vi "FL_DEC_split_3_and_prefilter_(online).vi"(0 "DEC input cluster":T4, 1 "Pre-filter params.":T1, 2 "Initialize? (F)":bool) -> (3 "Times":T3, 4 "TTLs":cluster{"TTL input":i16, "TTL output":i16}, 5 "Magnets coords":cluster{"X1":dbl, "Y1":dbl, "X2":dbl, "Y2":dbl}, 6 "Magnets coords raw":T2)   [LabVIEW 2018, in "Tracker.lvlib"]
uses:
  Tracker.lvlib
  Controls/CTL_Decoded_data_frame.ctl
  Controls/CTL_Pre-filter_params.ctl
  <vilib>/ptbypt/NI_PtbyPt.lvlib
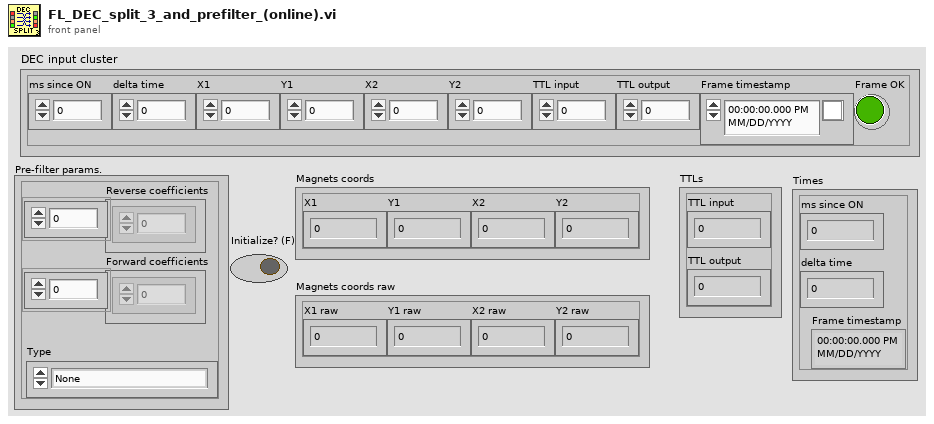
[diagram p1: front panel]
types:
  T1 = typedef "Tracker.lvlib/CTL_Pre-filter_params.ctl" = cluster{"Reverse coefficients":dbl[], "Forward coefficients":dbl[], "Type":enum16{"None", "FIR (PtbyPt)", "IIR (PtbyPt)"}}
  T2 = cluster{"X1 raw":dbl, "Y1 raw":dbl, "X2 raw":dbl, "Y2 raw":dbl}
  T3 = cluster{"ms since ON":u32, "delta time":u32, "Frame timestamp":timestamp}
  T4 = typedef "Tracker.lvlib/CTL_Decoded_data_frame.ctl" = cluster{"ms since ON":u32, "delta time":u32, "X1":sgl, "Y1":sgl, "X2":sgl, "Y2":sgl, "TTL input":i16, "TTL output":i16, "Frame timestamp":timestamp, "Frame OK":bool}
  T5 = cluster{"Filtered x":dbl, "Filtered x":dbl, "Filtered x":dbl, "Filtered x":dbl}
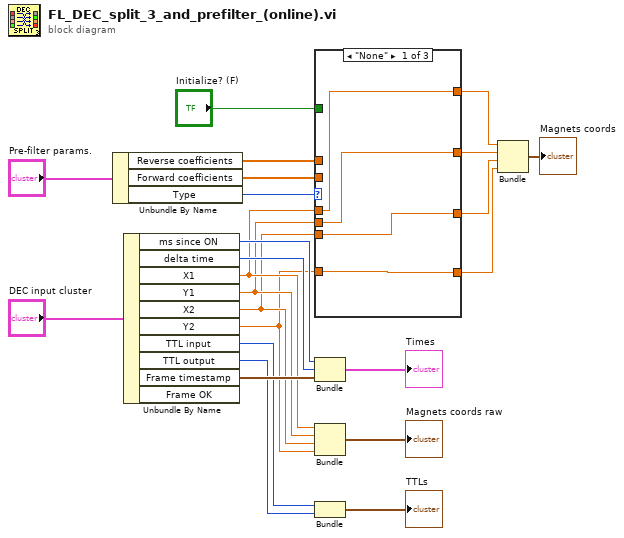
[diagram p0: block diagram]
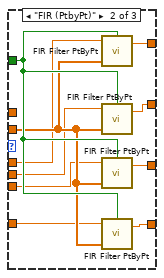
[diagram p2: hidden frame]
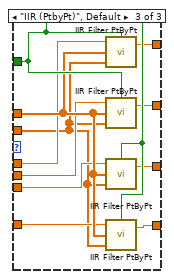
[diagram p3: hidden frame]
diagram:
  n1 = Unbundle By Name("Pre-filter params.") -> ("Reverse coefficients"=w12:dbl[], "Forward coefficients"=w11:dbl[], "Type"=w13:enum16{"None", "FIR (PtbyPt)", "IIR (PtbyPt)"})
  n2 = Unbundle By Name("DEC input cluster") -> ("ms since ON"=w22:u32, "delta time"=w21:u32, "X1"=w9:sgl, "Y1"=w8:sgl, "X2"=w7:sgl, "Y2"=w6:sgl, "TTL input"=w18:i16, "TTL output"=w17:i16, "Frame timestamp"=w20:timestamp)  [unwired: 1 out]
  n3 = case shown="\"None\"" w13 {
    tunnel: w12 -> [_ _ w47]
    tunnel: w11 -> [_ w36 w38]
    tunnel: "Initialize? (F)" -> [_ w37 w48]
    tunnel: w9 -> [w27 w35 w46]
    tunnel: w8 -> [w26 w33 w45]
    tunnel: w7 -> [w25 w31 w44]
    tunnel: w6 -> [w24 w29 w43]
    tunnel: [w27 w34 w42] -> w5
    tunnel: [w26 w32 w41] -> w4
    tunnel: [w25 w30 w40] -> w3
    tunnel: [w24 w28 w39] -> w2
    frame "None" {
    }
    frame "FIR (PtbyPt)" {
      n4 = call <vilib>:"FIR Filter PtByPt.vi"("initialize"=w37, "Forward Coefficients"=w36, "x"=w35) -> ("Filtered x"=w34:dbl)  [unwired: 1 in, 1 out]
      n5 = call <vilib>:"FIR Filter PtByPt.vi"("initialize"=w37, "Forward Coefficients"=w36, "x"=w33) -> ("Filtered x"=w32:dbl)  [unwired: 1 in, 1 out]
      n6 = call <vilib>:"FIR Filter PtByPt.vi"("initialize"=w37, "Forward Coefficients"=w36, "x"=w31) -> ("Filtered x"=w30:dbl)  [unwired: 1 in, 1 out]
      n7 = call <vilib>:"FIR Filter PtByPt.vi"("initialize"=w37, "Forward Coefficients"=w36, "x"=w29) -> ("Filtered x"=w28:dbl)  [unwired: 1 in, 1 out]
    }
    frame "IIR (PtbyPt)", Default {
      n8 = call <vilib>:"IIR Filter PtByPt.vi"("initialize"=w48, "Forward Coefficients"=w38, "Reverse Coefficients"=w47, "x"=w46) -> ("Filtered x"=w42:dbl)  [unwired: 1 out]
      n9 = call <vilib>:"IIR Filter PtByPt.vi"("initialize"=w48, "Forward Coefficients"=w38, "Reverse Coefficients"=w47, "x"=w45) -> ("Filtered x"=w41:dbl)  [unwired: 1 out]
      n10 = call <vilib>:"IIR Filter PtByPt.vi"("initialize"=w48, "Forward Coefficients"=w38, "Reverse Coefficients"=w47, "x"=w44) -> ("Filtered x"=w40:dbl)  [unwired: 1 out]
      n11 = call <vilib>:"IIR Filter PtByPt.vi"("initialize"=w48, "Forward Coefficients"=w38, "Reverse Coefficients"=w47, "x"=w43) -> ("Filtered x"=w39:dbl)  [unwired: 1 out]
    }
  }
  n12 = Bundle("ms since ON"=w22, "delta time"=w21, "Frame timestamp"=w20) -> (→"Times":T3)  [unwired: 1 in]
  n13 = Bundle("X1"=w9, "Y1"=w8, "X2"=w7, "Y2"=w6) -> (→"Magnets coords raw":cluster{"X1":sgl, "Y1":sgl, "X2":sgl, "Y2":sgl})  [unwired: 1 in]
  n14 = Bundle("TTL input"=w18, "TTL output"=w17) -> (→"TTLs":cluster{"TTL input":i16, "TTL output":i16})  [unwired: 1 in]
  n15 = Bundle("Filtered x"=w5, "Filtered x"=w4, "Filtered x"=w3, "Filtered x"=w2) -> (→"Magnets coords":T5)  [unwired: 1 in]
